vi "Instances search weekdays and weekdays.vi"(1 "Array in":string[](array[string])) -> (0 "Array out":string[](array[string]))   [LabVIEW 2015]
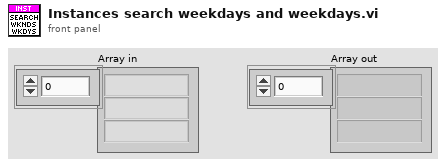
[diagram p1: front panel]
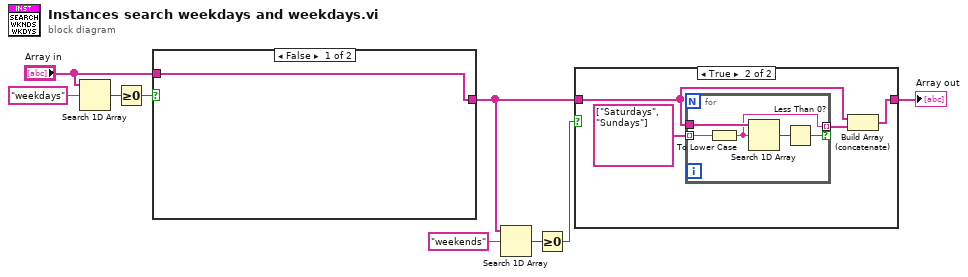
[diagram p0: block diagram]
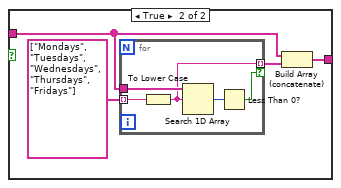
[diagram p3: hidden frame]
diagram:
  n1 = Search 1D Array(1D array="Array in", element="weekdays") -> (index of element=w2:i32)  [unwired: 1 in]
  n2 = Greater Or Equal To 0?(x=w2) -> (x >= 0?=w3:bool)
  n3 = case shown="False" w3 {
    tunnel: "Array in" -> [w10 w13]
    tunnel: [w10 w11] -> w9
    frame False {
    }
    frame True {
      n4 = for {
        tunnel: string[] ["Mondays", "Tuesdays", "Wednesdays", "Thursdays", "Fridays"] -> [w17] mode=indexing
        tunnel: w13 -> [w19]
        tunnel: [w15] -> w12 mode=indexing if=w16
        n5 = To Lower Case(string=w17) -> (all lower case string=w15:string)
        n6 = Search 1D Array(1D array=w19, element=w15) -> (index of element=w18:i32)  [unwired: 1 in]
        n7 = Less Than 0?(x=w18) -> (x < 0?=w16:bool)
      }
      n8 = Build Array (concatenate)(w13, w12) -> (w11:string[])
    }
  }
  n9 = Search 1D Array(1D array=w9, element="weekends") -> (index of element=w6:i32)  [unwired: 1 in]
  n10 = Greater Or Equal To 0?(x=w6) -> (x >= 0?=w5:bool)
  n11 = case shown="True" w5 {
    tunnel: w9 -> [w20 w23]
    tunnel: [w20 w21] -> w8
    frame False {
    }
    frame True {
      n12 = for {
        tunnel: string[] ["Saturdays", "Sundays"] -> [w27] mode=indexing
        tunnel: w23 -> [w29]
        tunnel: [w25] -> w22 mode=indexing if=w26
        n13 = To Lower Case(string=w27) -> (all lower case string=w25:string)
        n14 = Search 1D Array(1D array=w29, element=w25) -> (index of element=w28:i32)  [unwired: 1 in]
        n15 = Less Than 0?(x=w28) -> (x < 0?=w26:bool)
      }
      n16 = Build Array (concatenate)(w23, w22) -> (w21:string[])
    }
  }
  "Array out" <- w8
